vi "Lab Panel V4.82.vi"() -> ()   [LabVIEW 2013] (continued)
          n31 = local read "Fail Loops"() -> (w22:dbl)
          n32 = Bundle("SET LAB01-1"=w59, "SET LAB01-2"=w60, "SET LAB02-1"=w61, "SET LAB02-2"=w62, "SET LAB03-1"=w63, "SET LAB03-2"=w64, "SET LAB04-1"=w68, "SET LAB04-2"=w67, "SET LAB05-1"=w66, "SET LAB05-2"=w65, "Network Directory"=w35, "C drive data root dir"=w33, "RATE (Hz)"=w32, "SAMPLES"=w31, "Select COM port"=w27, "Temp Delay Lps"=w26, "Temp Value"=w25, "Fail Loops"=w22, "Temp Test Cal"=w20, "Set Temp Lps"=w19) -> (w52:T21)  [unwired: 1 in]
          n33 = String To Path(string="c:\\crabtree\\Set Up\\") -> (path=w56:path)
          n34 = Build Path(base path=w56, name or relative path="settings.bin") -> (appended path=w54:path)
          n35 = Create Folder(path (use dialog)=w56) -> (error out=w58:errorcluster)  [unwired: 2 in, 2 out]
          n36 = call <vilib>:"Clear Errors.vi"("error in (no error)"=w58) -> ()  [unwired: 6 in, 1 out]
          n37 = Open/Create/Replace File(file path (use dialog)=w54) -> (refnum out=w51:refnum<file>, error out=w53:errorcluster)  [unwired: 5 in, 1 out]
          n38 = Read from Binary File(5:w52, 8:w53, 11:w51) -> (0:w48:errorcluster, 2:w50:T21, 3:w49:refnum<file>)  [unwired: 3 in, 1 out]
          n39 = Unbundle(w50) -> ("SET LAB01-1"=w46:T5, "SET LAB01-2"=w45:T5, "SET LAB02-1"=w44:T5, "SET LAB02-2"=w43:T5, "SET LAB03-1"=w42:T5, "SET LAB03-2"=w41:T5, "SET LAB04-1"=w40:T5, "SET LAB04-2"=w39:T5, "SET LAB05-1"=w38:T5, "SET LAB05-2"=w37:T5, "Network Directory"=w36:path, "C drive data root dir"=w34:path, "RATE (Hz)"=w29:dbl, "SAMPLES"=w30:dbl, "Select COM port"=w28:refnum<visa-resource-name>, "Temp Delay Lps"=w24:dbl, "Temp Value"=w23:dbl, "Fail Loops"=w21:dbl, "Temp Test Cal"=w18:dbl, "Set Temp Lps"=w17:dbl)
          n40 = Close File(refnum=w49, error in=w48) -> (error out=w47:errorcluster)  [unwired: 1 out]
          n41 = local write "data file error"(w47) -> ()
          n42 = local write "Temp Test Cal"(w18) -> ()
          n43 = local write "Set Temp Lps"(w17) -> ()
          n44 = local write "Fail Loops"(w21) -> ()
          n45 = local write "Temp Delay Lps"(w24) -> ()
          n46 = local write "C drive data root dir"(w34) -> ()
          n47 = local write "Temp Value"(w23) -> ()
          n48 = local write "Select COM port"(w28) -> ()
          n49 = local write "Network Directory"(w36) -> ()
          n50 = local write "SAMPLES"(w30) -> ()
          n51 = local write "RATE (Hz)"(w29) -> ()
          n52 = local write "SET LAB04-2"(w39) -> ()
          n53 = local write "SET LAB05-1"(w38) -> ()
          n54 = local write "SET LAB04-1"(w40) -> ()
          n55 = local write "SET LAB05-2"(w37) -> ()
          n56 = local write "SET LAB02-1"(w44) -> ()
          n57 = local write "SET LAB02-2"(w43) -> ()
          n58 = local write "SET LAB03-1"(w42) -> ()
          n59 = local write "SET LAB03-2"(w41) -> ()
          n60 = local write "SET LAB01-1"(w46) -> ()
          n61 = local write "SET LAB01-2"(w45) -> ()
        }
        frame #3 {
          # "get last saved jig cycles value from file"
          n62 = String To Path(string="c:\\crabtree\\Jig Cycles\\") -> (path=w78:path)
          n63 = Build Path(base path=w78, name or relative path="jigcycles.bin") -> (appended path=w76:path)
          n64 = Create Folder(path (use dialog)=w78) -> (error out=w80:errorcluster)  [unwired: 2 in, 2 out]
          n65 = call <vilib>:"Clear Errors.vi"("error in (no error)"=w80) -> ()  [unwired: 6 in, 1 out]
          n66 = Open/Create/Replace File(file path (use dialog)=w76) -> (refnum out=w74:refnum<file>, error out=w75:errorcluster)  [unwired: 5 in, 1 out]
          n67 = Read from Binary File(5:T10 {"LAB01-1"=0.0, "LAB01-2"=0.0, "LAB02-1"=0.0, "LAB02-2"=0.0, "LAB03-1"=0.0, "LAB03-2"=0.0, "LAB04-1"=0.0, "LAB04-2"=0.0, "LAB05-1"=0.0, "LAB05-2"=0.0} ("JIG RELAY CYCLES"), 8:w75, 11:w74) -> (0:w72:errorcluster, 2:w69:T10, 3:w73:refnum<file>)  [unwired: 3 in, 1 out]
          n68 = local write "JIG RELAY CYCLES"(w69) -> ()
          n69 = Close File(refnum=w73, error in=w72) -> (error out=w71:errorcluster)  [unwired: 1 out]
          n70 = local write "data file error"(w71) -> ()
        }
        frame #4 {
          # "get mail settings"
          n71 = local read "Auto Mail Send"() -> (w84:bool)
          n72 = local read "MAIL SETTINGS"() -> (w88:T7)
          n73 = String To Path(string="c:\\crabtree\\Set Up\\") -> (path=w96:path)
          n74 = Build Path(base path=w96, name or relative path="mail.bin") -> (appended path=w94:path)
          n75 = Create Folder(path (use dialog)=w96) -> (error out=w98:errorcluster)  [unwired: 2 in, 2 out]
          n76 = Bundle("MAIL SETTINGS"=w88, "Auto Mail Send"=w84, "") -> (w87:T22)  [unwired: 1 in]
          n77 = call <vilib>:"Clear Errors.vi"("error in (no error)"=w98) -> ()  [unwired: 6 in, 1 out]
          n78 = Open/Create/Replace File(file path (use dialog)=w94) -> (refnum out=w92:refnum<file>, error out=w93:errorcluster)  [unwired: 5 in, 1 out]
          n79 = Read from Binary File(5:w87, 8:w93, 11:w92) -> (0:w90:errorcluster, 2:w86:T22, 3:w91:refnum<file>)  [unwired: 3 in, 1 out]
          n80 = Unbundle(w86) -> ("MAIL SETTINGS"=w85:T7, "Auto Mail Send"=w83:bool, w82:string)
          n81 = local write "TO (string):"(w82) -> ()
          n82 = local write "Auto Mail Send"(w83) -> ()
          n83 = local write "MAIL SETTINGS"(w85) -> ()
          n84 = Close File(refnum=w91, error in=w90) -> (error out=w89:errorcluster)  [unwired: 1 out]
          n85 = local write "data file error"(w89) -> ()
        }
        frame #5 {
          # "set display status if blank"
          n86 = local read "DISP LAB03-2"() -> (w128:T4)
          n87 = local read "DISP LAB03-1"() -> (w135:T4)
          n88 = local read "DISP LAB02-2"() -> (w142:T4)
          n89 = local read "DISP LAB01-2"() -> (w155:T4)
          n90 = local read "DISP LAB01-1"() -> (w164:T4)
          n91 = local read "DISP LAB02-1"() -> (w149:T4)
          n92 = Unbundle(w128) -> ("STATUS"=w130:string)  [unwired: 2 out]
          n93 = Unbundle(w135) -> ("STATUS"=w137:string)  [unwired: 2 out]
          n94 = Unbundle(w142) -> ("STATUS"=w144:string)  [unwired: 2 out]
          n95 = Unbundle(w149) -> ("STATUS"=w151:string)  [unwired: 2 out]
          n96 = Unbundle(w155) -> ("STATUS"=w158:string)  [unwired: 2 out]
          n97 = Unbundle(w164) -> ("STATUS"=w165:string)  [unwired: 2 out]
          n98 = Equal?(x="", y=w130) -> (x = y?=w132:bool)
          n99 = Equal?(x="", y=w137) -> (x = y?=w139:bool)
          n100 = Equal?(x="", y=w144) -> (x = y?=w146:bool)
          n101 = Equal?(x="", y=w151) -> (x = y?=w153:bool)
          n102 = Equal?(x="", y=w158) -> (x = y?=w160:bool)
          n103 = Equal?(x="", y=w165) -> (x = y?=w167:bool)
          n104 = Select(t="STOP", s=w132, f=w130) -> (s? t:f=w129:string)
          n105 = Select(t="STOP", s=w139, f=w137) -> (s? t:f=w136:string)
          n106 = Select(t="STOP", s=w146, f=w144) -> (s? t:f=w143:string)
          n107 = Select(t="STOP", s=w153, f=w151) -> (s? t:f=w150:string)
          n108 = Select(t="STOP", s=w160, f=w158) -> (s? t:f=w157:string)
          n109 = Select(t="STOP", s=w167, f=w165) -> (s? t:f=w163:string)
          n110 = Bundle(cluster=w128, "STATUS"=w129) -> (w127:T4)  [unwired: 2 in]
          n111 = Bundle(cluster=w135, "STATUS"=w136) -> (w134:T4)  [unwired: 2 in]
          n112 = Bundle(cluster=w142, "STATUS"=w143) -> (w141:T4)  [unwired: 2 in]
          n113 = Bundle(cluster=w149, "STATUS"=w150) -> (w148:T4)  [unwired: 2 in]
          n114 = Bundle(cluster=w155, "STATUS"=w157) -> (w156:T4)  [unwired: 2 in]
          n115 = Bundle(cluster=w164, "STATUS"=w163) -> (w162:T4)  [unwired: 2 in]
          n116 = local write "DISP LAB01-2"(w156) -> ()
          n117 = local write "DISP LAB01-1"(w162) -> ()
          n118 = local write "DISP LAB02-1"(w148) -> ()
          n119 = local write "DISP LAB03-1"(w134) -> ()
          n120 = local write "DISP LAB02-2"(w141) -> ()
          n121 = local write "DISP LAB03-2"(w127) -> ()
          n122 = local read "DISP LAB05-2"() -> (w100:T4)
          n123 = local read "DISP LAB05-1"() -> (w107:T4)
          n124 = local read "DISP LAB04-2"() -> (w109:T4)
          n125 = local read "DISP LAB04-1"() -> (w111:T4)
          n126 = Unbundle(w100) -> ("STATUS"=w102:string)  [unwired: 2 out]
          n127 = Unbundle(w107) -> ("STATUS"=w113:string)  [unwired: 2 out]
          n128 = Unbundle(w109) -> ("STATUS"=w118:string)  [unwired: 2 out]
          n129 = Unbundle(w111) -> ("STATUS"=w123:string)  [unwired: 2 out]
          n130 = Equal?(x="", y=w102) -> (x = y?=w104:bool)
          n131 = Equal?(x="", y=w113) -> (x = y?=w115:bool)
          n132 = Equal?(x="", y=w118) -> (x = y?=w120:bool)
          n133 = Equal?(x="", y=w123) -> (x = y?=w125:bool)
          n134 = Select(t="STOP", s=w104, f=w102) -> (s? t:f=w101:string)
          n135 = Select(t="STOP", s=w115, f=w113) -> (s? t:f=w112:string)
          n136 = Select(t="STOP", s=w120, f=w118) -> (s? t:f=w117:string)
          n137 = Select(t="STOP", s=w125, f=w123) -> (s? t:f=w122:string)
          n138 = Bundle(cluster=w100, "STATUS"=w101) -> (w99:T4)  [unwired: 2 in]
          n139 = Bundle(cluster=w107, "STATUS"=w112) -> (w106:T4)  [unwired: 2 in]
          n140 = Bundle(cluster=w109, "STATUS"=w117) -> (w108:T4)  [unwired: 2 in]
          n141 = Bundle(cluster=w111, "STATUS"=w122) -> (w110:T4)  [unwired: 2 in]
          n142 = local write "DISP LAB05-2"(w99) -> ()
          n143 = local write "DISP LAB05-1"(w106) -> ()
          n144 = local write "DISP LAB04-1"(w110) -> ()
          n145 = local write "DISP LAB04-2"(w108) -> ()
        }
        frame #6 {
          # "initialise analog input express vi's"
          n146 = for {
            N: 2.0 -> [_]
            n147 = call "sub vi - analog 1st setup v1.vi"() -> ("error out"=w171:errorcluster)  [unwired: 11 in, 4 out]
            n148 = Unbundle(w171) -> ("status"=w170:bool)  [unwired: 2 out]
            n149 = local write "simulate"(w170) -> ()
          }
        }
        frame #7 {
          # "get initial temperature values"
          n150 = stacked-sequence {
            frame #0 {
              w178 = TRUE
              n151 = call "sub vi - GET ALL TEMP v4.vi"("LA01-EN"=w178, "LA02-EN"=w178, "LA03-EN"=w178, "LA04-EN"=w178, "LA05-EN"=w178, "Gen Cal Value"=1) -> ("LA01 TEMP"=w176:T23, "LA02 TEMP"=w175:T23, "LA03 TEMP"=w174:T23, "LA04 TEMP"=w173:T23, "LA05 TEMP"=w172:T23)  [unwired: 4 in, 1 out]
              n152 = local write "LAB01 TEMP"(w176) -> ()
              n153 = local write "LAB02 TEMP"(w175) -> ()
              n154 = local write "LAB04 TEMP"(w173) -> ()
              n155 = local write "LAB03 TEMP"(w174) -> ()
              n156 = local write "LAB05 TEMP"(w172) -> ()
            }
            frame #1 {
              w179 = 0
              n157 = local read "LAB01 TEMP"() -> (w185:T14)
              n158 = Unbundle By Name(w185) -> ("T1 Live"=w184:dbl, "T1 Neut"=w183:dbl, "T2 Live"=w182:dbl, "T2 Neut"=w181:dbl)  [unwired: 2 out]
              n159 = local read "TEMP LA01"() -> (w186:T11)
              n160 = Bundle By Name(cluster=w186, "TL-1"=w184, "TN-1"=w183, "TL-2"=w182, "TN-2"=w181, "TL -1COUNT"=w179, "TN-1 COUNT"=w179, "TL-2 COUNT"=w179, "TN-2 COUNT"=w179) -> (w180:T11)
              n161 = local write "TEMP LA01"(w180) -> ()
            }
            frame #2 {
              w187 = 0
              n162 = local read "LAB02 TEMP"() -> (w193:T14)
              n163 = Unbundle By Name(w193) -> ("T1 Live"=w192:dbl, "T1 Neut"=w191:dbl, "T2 Live"=w190:dbl, "T2 Neut"=w189:dbl)  [unwired: 2 out]
              n164 = local read "TEMP LA02"() -> (w194:T11)
              n165 = Bundle By Name(cluster=w194, "TL-1"=w192, "TN-1"=w191, "TL-2"=w190, "TN-2"=w189, "TL -1COUNT"=w187, "TN-1 COUNT"=w187, "TL-2 COUNT"=w187, "TN-2 COUNT"=w187) -> (w188:T11)
              n166 = local write "TEMP LA02"(w188) -> ()
            }
            frame #3 {
              w195 = 0
              n167 = local read "LAB03 TEMP"() -> (w201:T14)
              n168 = Unbundle By Name(w201) -> ("T1 Live"=w200:dbl, "T1 Neut"=w199:dbl, "T2 Live"=w198:dbl, "T2 Neut"=w197:dbl)  [unwired: 2 out]
              n169 = local read "TEMP LA03"() -> (w202:T11)
              n170 = Bundle By Name(cluster=w202, "TL-1"=w200, "TN-1"=w199, "TL-2"=w198, "TN-2"=w197, "TL -1COUNT"=w195, "TN-1 COUNT"=w195, "TL-2 COUNT"=w195, "TN-2 COUNT"=w195) -> (w196:T11)
              n171 = local write "TEMP LA03"(w196) -> ()
            }
            frame #4 {
              w203 = 0
              n172 = local read "LAB04 TEMP"() -> (w209:T14)
              n173 = Unbundle By Name(w209) -> ("T1 Live"=w208:dbl, "T1 Neut"=w207:dbl, "T2 Live"=w206:dbl, "T2 Neut"=w205:dbl)  [unwired: 2 out]
              n174 = local read "TEMP LA04"() -> (w210:T11)
              n175 = Bundle By Name(cluster=w210, "TL-1"=w208, "TN-1"=w207, "TL-2"=w206, "TN-2"=w205, "TL -1COUNT"=w203, "TN-1 COUNT"=w203, "TL-2 COUNT"=w203, "TN-2 COUNT"=w203) -> (w204:T11)
              n176 = local write "TEMP LA04"(w204) -> ()
            }
            frame #5 {
              w211 = 0
              n177 = local read "LAB05 TEMP"() -> (w217:T14)
              n178 = Unbundle By Name(w217) -> ("T1 Live"=w216:dbl, "T1 Neut"=w215:dbl, "T2 Live"=w214:dbl, "T2 Neut"=w213:dbl)  [unwired: 2 out]
              n179 = local read "TEMP LA05"() -> (w218:T11)
              n180 = Bundle By Name(cluster=w218, "TL-1"=w216, "TN-1"=w215, "TL-2"=w214, "TN-2"=w213, "TL -1COUNT"=w211, "TN-1 COUNT"=w211, "TL-2 COUNT"=w211, "TN-2 COUNT"=w211) -> (w212:T11)
              n181 = local write "TEMP LA05"(w212) -> ()
            }
          }
        }
        frame #8 {
          # "enable front panel, all settings done"
          n182 = property on="Tab Control 2" class="TabCtl (strict)"("DisabledEnum"=T15."Enabled" ("Disabled")) -> ()  [unwired: 2 in, 2 out]
          n183 = property on="Tab Control 2" class="TabCtl (strict)"("Value"=0) -> ()  [unwired: 2 in, 2 out]
        }
        frame #9 {
          # "check network directory valid"
          n184 = while {
            stop <- w223 continue-if-true
            w221 = TRUE
            n185 = local read "Network Directory"() -> (w225:path)
            n186 = property on="Tab Control 2" class="TabCtl (strict)"("Value"=5) -> ()  [unwired: 2 in, 2 out]
            n187 = File/Directory Info(path=w225) -> (error out=w226:errorcluster)  [unwired: 1 in, 6 out]
            n188 = Unbundle(w226) -> ("status"=w223:bool)  [unwired: 2 out]
            n189 = case shown="True" w223 {
              frame False {
                n190 = local write "Message"("") -> ()
              }
              frame True {
                "Message" <- "NETWORK DIRECTORY NOT FOUND!!!!"
              }
            }
            n191 = property on="Message" class="Str"("Text.TextColor"=u32 16711680) -> ()  [unwired: 2 in, 2 out]
            n192 = property on="Network Directory" class="Path"("Blinking"=w221) -> ()  [unwired: 2 in, 2 out]
            n193 = property on="Message" class="Str"("Blinking"=w221) -> ()  [unwired: 2 in, 2 out]
          }
        }
        frame #10 {
          w229 = FALSE
          n194 = property on="Message" class="Str"("Blinking"=w229) -> ()  [unwired: 2 in, 2 out]
          n195 = property on="Network Directory" class="Path"("Blinking"=w229) -> ()  [unwired: 2 in, 2 out]
          n196 = property on="Tab Control 2" class="TabCtl (strict)"("Value"=0) -> ()  [unwired: 2 in, 2 out]
        }
      }
    }
    frame #2 {
      n197 = node-c288("loop  delay(mS)") -> (w233:T16)  [unwired: 3 in]
      n198 = timed-loop {
        timing: w233 -> [_]
        timing-out: [_] -> w232
        i -> [w255]
        stop <- "stop" stop-if-true
        n199 = node-c288() -> ()  [unwired: 1 in, 1 out]
        n200 = local read "SELECT LAB05-2"() -> (w235:T3)
        n201 = local read "SELECT LAB05-1"() -> (w236:T3)
        n202 = local read "SELECT LAB04-2"() -> (w237:T3)
        n203 = local read "SELECT LAB03-1"() -> (w240:T3)
        n204 = local read "SELECT LAB02-2"() -> (w241:T3)
        n205 = local read "SELECT LAB01-1"() -> (w244:T3)
        n206 = local read "SELECT LAB03-2"() -> (w239:T3)
        n207 = local read "SELECT LAB01-2"() -> (w243:T3)
        n208 = local read "SELECT LAB04-1"() -> (w238:T3)
        n209 = local read "SELECT LAB02-1"() -> (w242:T3)
        n210 = local read "run lab03-2"() -> (w249:bool)
        n211 = local read "run lab04-1"() -> (w248:bool)
        n212 = local read "run lab05-1"() -> (w246:bool)
        n213 = local read "run lab04-2"() -> (w247:bool)
        n214 = local read "run lab05-2"() -> (w245:bool)
        n215 = local read "run lab03-1"() -> (w250:bool)
        n216 = local read "run lab02-2"() -> (w251:bool)
        n217 = local read "run lab02-1"() -> (w252:bool)
        n218 = local read "run lab01-1"() -> (w254:bool)
        n219 = local read "run lab01-2"() -> (w253:bool)
        n220 = stacked-sequence {
          seq-local: [_ w319 _ _ _ _ _ _ _ _ _ _ _ _ _ _ _ _ _ _] -> [_ _ _ _ _ w1926 _ _ _ _ _ _ _ _ _ _ _ _ _ _]
          seq-local: [_ w318 _ _ _ _ _ _ _ _ _ _ _ _ _ _ _ _ _ _] -> [_ _ _ _ _ w1925 _ _ _ _ _ _ _ _ _ _ _ _ _ _]
          seq-local: [_ w305 _ _ _ _ _ _ _ _ _ _ _ _ _ _ _ _ _ _] -> [_ _ _ _ _ w1924 _ _ _ _ _ _ _ _ _ _ _ _ _ _]
          seq-local: [_ w304 _ _ _ _ _ _ _ _ _ _ _ _ _ _ _ _ _ _] -> [_ _ _ _ _ w1923 _ _ _ _ _ _ _ _ _ _ _ _ _ _]
          seq-local: [_ w303 _ _ _ _ _ _ _ _ _ _ _ _ _ _ _ _ _ _] -> [_ _ _ _ _ w1922 _ _ _ _ _ _ _ _ _ _ _ _ _ _]
          seq-local: [_ w302 _ _ _ _ _ _ _ _ _ _ _ _ _ _ _ _ _ _] -> [_ _ _ _ _ w1921 _ _ _ _ _ _ _ _ _ _ _ _ _ _]
          seq-local: [_ w301 _ _ _ _ _ _ _ _ _ _ _ _ _ _ _ _ _ _] -> [_ _ _ _ _ w1920 _ _ _ _ _ _ _ _ _ _ _ _ _ _]
          seq-local: [_ w300 _ _ _ _ _ _ _ _ _ _ _ _ _ _ _ _ _ _] -> [_ _ _ _ _ w1919 _ _ _ _ _ _ _ _ _ _ _ _ _ _]
          seq-local: [_ w299 _ _ _ _ _ _ _ _ _ _ _ _ _ _ _ _ _ _] -> [_ _ _ _ _ w1918 _ _ _ _ _ _ _ _ _ _ _ _ _ _]
          seq-local: [_ w298 _ _ _ _ _ _ _ _ _ _ _ _ _ _ _ _ _ _] -> [_ _ _ _ _ w1917 _ _ _ _ _ _ _ _ _ _ _ _ _ _]
          tunnel: w254 -> [_ _ w335 w572 w1516 w1946 w2256 w2501 _ _ _ _ w2904 _ w3832 _ _ w4115 w4418 w4591]
          tunnel: w253 -> [_ _ w334 w570 w1515 w1945 w2257 w2500 _ _ _ _ w2903 _ w3830 _ _ w4114 w4417 w4589]
          tunnel: w252 -> [_ _ w333 w568 w1514 w1944 w2255 w2499 _ _ _ _ w2902 _ w3828 _ _ w4113 w4416 _]
          tunnel: w251 -> [_ _ w332 w566 w1513 w1943 w2254 w2498 _ _ _ _ w2901 _ w3826 _ _ w4112 w4415 _]
          tunnel: w250 -> [_ _ w331 w564 w1512 w1942 w2253 w2497 _ _ _ _ w2900 _ w3824 _ _ w4111 w4414 _]
          tunnel: w249 -> [_ _ w330 w562 w1511 w1941 w2252 w2496 _ _ _ _ w2899 _ w3822 _ _ w4110 w4413 _]
          tunnel: w248 -> [_ _ w329 w560 w1510 w1940 w2251 w2495 _ _ _ _ w2898 _ w3820 _ _ w4109 w4412 _]
          tunnel: w247 -> [_ _ w328 w558 w1509 w1939 w2250 w2494 _ _ _ _ w2897 _ w3818 _ _ w4108 w4411 _]
          tunnel: w246 -> [_ _ w327 w556 w1508 w1938 w2249 w2493 _ _ _ _ w2896 _ w3816 _ _ w4107 w4410 _]
          tunnel: w245 -> [_ _ w326 w554 w1507 w1937 w2248 w2492 _ _ _ _ w2895 _ w3814 _ _ w4106 w4409 _]
          tunnel: w244 -> [_ _ _ w571 w1506 w1936 _ _ _ _ _ _ _ _ w3834 _ _ _ _ _]
          tunnel: w243 -> [_ _ _ w569 w1505 w1935 _ _ _ _ _ _ _ _ w3829 _ _ _ _ _]
          tunnel: w242 -> [_ _ _ w567 w1504 w1934 _ _ _ _ _ _ _ _ w3827 _ _ _ _ _]
          tunnel: w241 -> [_ _ _ w565 w1503 w1933 _ _ _ _ _ _ _ _ w3825 _ _ _ _ _]
          tunnel: w240 -> [_ _ _ w563 w1502 w1932 _ _ _ _ _ _ _ _ w3823 _ _ _ _ _]
          tunnel: w239 -> [_ _ _ w561 w1501 w1931 _ _ _ _ _ _ _ _ w3821 _ _ _ _ _]
          tunnel: w238 -> [_ _ _ w559 w1500 w1930 _ _ _ _ _ _ _ _ w3819 _ _ _ _ _]
          tunnel: w237 -> [_ _ _ w557 w1499 w1929 _ _ _ _ _ _ _ _ w3817 _ _ _ _ _]
          tunnel: w236 -> [_ _ _ w555 w1498 w1928 _ _ _ _ _ _ _ _ w3815 _ _ _ _ _]
          tunnel: w235 -> [_ _ _ w553 w1497 w1927 _ _ _ _ _ _ _ _ w3813 _ _ _ _ _]
          frame #0 {
            w261 = FALSE
            w266 = 0.5
            # "set up cycle control"
            n221 = local read "jig cycle"() -> (w265:dbl)
            n222 = local read "Temp Loops"() -> (w259:dbl)
            n223 = Divide(x="JIG ON TIME (S)", y=w266) -> (x/y=→"on loops":dbl)
            n224 = Divide(x="JIG OFF TIME (S)", y=w266) -> (x/y=→"off loops":dbl)
            n225 = Increment(x=w265) -> (x+1=w264:dbl)
            n226 = local write "TEMP update"(w261) -> ()
            n227 = Increment(x=w259) -> (x+1=w258:dbl)
            n228 = local write "AI update"(w261) -> ()
            n229 = local write "Temp Loops"(w258) -> ()
            n230 = local write "jig cycle"(w264) -> ()
            n231 = event shown="[1] \"ADMIN PAGE\": Value Change" {
              selector: _ -> [_ _]
              dyn-events: _ -> [_ _]
              timeout: 10 -> [_ _]
              event Timeout {
                n232 = event-data() -> ()  [unwired: 1 in, 3 out]
              }
              event "ADMIN PAGE": Value Change {
                n233 = event-data() -> ()  [unwired: 1 in, 6 out]
                n234 = stacked-sequence {
                  seq-local: [_ w270 _] -> [_ _ w271]
                  frame #0 {
                    n235 = global write "Global 1.vi" "password"("9999") -> ()
                  }
                  frame #1 {
                    n236 = call "sub vi - password 1.vi"() -> ("RESULT"=w270:bool)  [unwired: 11 in]
                  }
                  frame #2 {
                    w273 = FALSE
                    n237 = property on="Tab Control 2" class="TabCtl (strict)"() -> ("Pages"=w277:refnum<vi>[])  [unwired: 2 in, 2 out]
                    n238 = Select(t=TRUE, s=w271, f=w273) -> (s? t:f=w272:bool)
                    n239 = Index Array(array=w277, index=9) -> (element=w275:refnum<vi>)
                    n240 = property class="Page"(reference=w275, "PageVis"=w272) -> ()  [unwired: 1 in, 2 out]
                    n241 = local write "ADMIN PAGE"(w273) -> ()
                  }
                }
              }
            }
          }
          frame #1 {
            w315 = 60.0
            # "convert temperature rise minutes to cycles"
            n242 = local read "SET LAB05-2"() -> (w279:T5)
            n243 = local read "SET LAB05-1"() -> (w281:T5)
            n244 = local read "SET LAB04-2"() -> (w283:T5)
            n245 = local read "SET LAB01-1"() -> (w297:T5)
            n246 = local read "SET LAB01-2"() -> (w295:T5)
            n247 = local read "SET LAB02-2"() -> (w291:T5)
            n248 = local read "SET LAB04-1"() -> (w285:T5)
            n249 = local read "SET LAB03-1"() -> (w289:T5)
            n250 = local read "SET LAB03-2"() -> (w287:T5)
            n251 = local read "SET LAB02-1"() -> (w293:T5)
            n252 = local read "JIG OFF TIME (S)"() -> (w320:dbl)
            n253 = local read "JIG ON TIME (S)"() -> (w321:dbl)
            n254 = Unbundle(w279) -> ("T-RISE mins"=w278:dbl)  [unwired: 4 out]
            n255 = Unbundle(w281) -> ("T-RISE mins"=w280:dbl)  [unwired: 4 out]
            n256 = Unbundle(w297) -> ("T-RISE mins"=w296:dbl)  [unwired: 4 out]
            n257 = Unbundle(w283) -> ("T-RISE mins"=w282:dbl)  [unwired: 4 out]
            n258 = Unbundle(w295) -> ("T-RISE mins"=w294:dbl)  [unwired: 4 out]
            n259 = Unbundle(w293) -> ("T-RISE mins"=w292:dbl)  [unwired: 4 out]
            n260 = Unbundle(w285) -> ("T-RISE mins"=w284:dbl)  [unwired: 4 out]
            n261 = Unbundle(w291) -> ("T-RISE mins"=w290:dbl)  [unwired: 4 out]
            n262 = Unbundle(w287) -> ("T-RISE mins"=w286:dbl)  [unwired: 4 out]
            n263 = Unbundle(w289) -> ("T-RISE mins"=w288:dbl)  [unwired: 4 out]
            n264 = Add(x=w321, y=w320) -> (x+y=w314:dbl)
            n265 = Multiply(x=w315, y=w286) -> (x*y=w310:dbl)
            n266 = Multiply(x=w315, y=w284) -> (x*y=w309:dbl)
            n267 = Multiply(x=w315, y=w282) -> (x*y=w308:dbl)
            n268 = Multiply(x=w315, y=w280) -> (x*y=w307:dbl)
            n269 = Multiply(x=w315, y=w278) -> (x*y=w306:dbl)
            n270 = Multiply(x=w315, y=w294) -> (x*y=w316:dbl)
            n271 = Multiply(x=w315, y=w288) -> (x*y=w311:dbl)
            n272 = Multiply(x=w315, y=w296) -> (x*y=w317:dbl)
            n273 = Multiply(x=w315, y=w292) -> (x*y=w313:dbl)
            n274 = Multiply(x=w315, y=w290) -> (x*y=w312:dbl)
            n275 = Divide(x=w307, y=w314) -> (x/y=w299:dbl)
            n276 = Divide(x=w308, y=w314) -> (x/y=w300:dbl)
            n277 = Divide(x=w309, y=w314) -> (x/y=w301:dbl)
            n278 = Divide(x=w306, y=w314) -> (x/y=w298:dbl)
            n279 = Divide(x=w311, y=w314) -> (x/y=w303:dbl)
            n280 = Divide(x=w317, y=w314) -> (x/y=w319:dbl)
            n281 = Divide(x=w316, y=w314) -> (x/y=w318:dbl)
            n282 = Divide(x=w313, y=w314) -> (x/y=w305:dbl)
            n283 = Divide(x=w312, y=w314) -> (x/y=w304:dbl)
            n284 = Divide(x=w310, y=w314) -> (x/y=w302:dbl)
          }
          frame #2 {
            # "control cycle loops"
            n285 = local read "JIG OFF TIME (S)"() -> (w324:dbl)
            n286 = local read "JIG ON TIME (S)"() -> (w323:dbl)
